vi "Demo.vi"() -> ()   [LabVIEW 2019]
uses:
  IO_VI/IOCtrl/Ctrl/IO Card_Type.ctl
panel:
  in  "IOType":enum16{"InputAndOutput", "Input", "OutPut"}(ring)
  in  "stop":bool
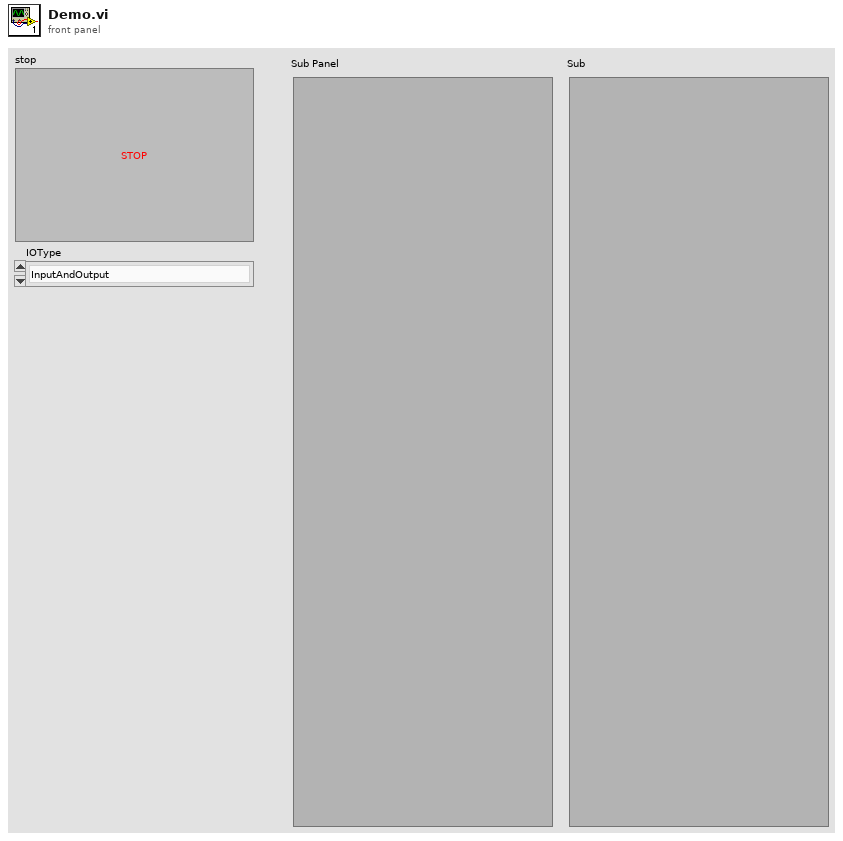
[diagram p1: front panel]
types:
  T1 = typedef "IO Card_Type.ctl" = enum16{"None", "Unidaq32", "6480", "2410C-64", "Zan", "DMC1000B"}
  T2 = typedef "LVPointTypeDef.ctl" = cluster{"Horizontal":i16, "Vertical":i16}
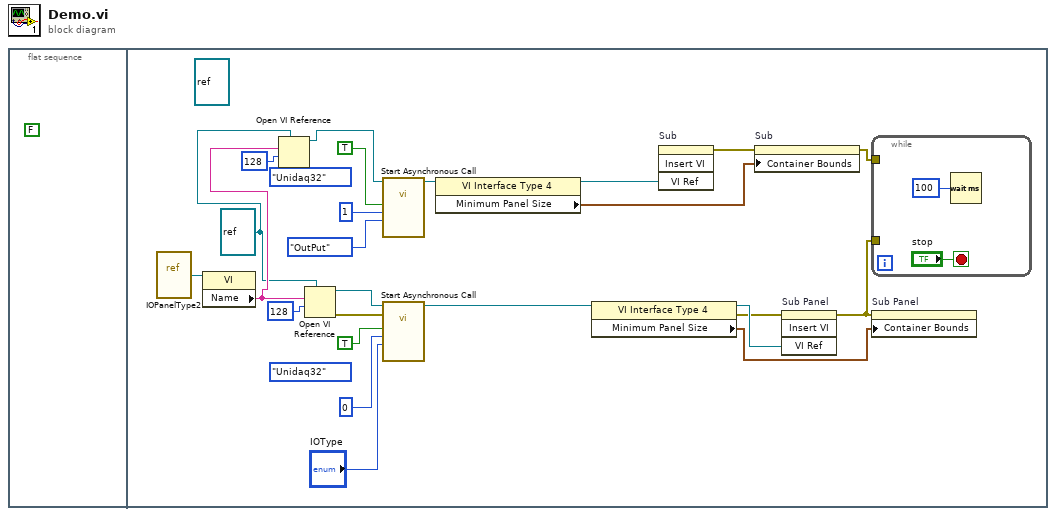
[diagram p0: block diagram]
diagram:
  n1 = flat-sequence {
    frame #0 {
      (unwired) FALSE ("Stopflg")
    }
    frame #1 {
      (unwired) refnum<vi> refnum ("reference out")
      (unwired) IO_Card_Type."Unidaq32" ("Card_Type")
      (unwired) IO_Card_Type."Unidaq32" ("Card_Type")
      w1 = refnum<vi> refnum ("reference out")
      n2 = vi-ref "IOPanelType2.vi"() -> (w23:refnum<vi>)
      n3 = property class="VI"(reference=w23) -> ("Name"=w3:string)  [unwired: 1 in, 2 out]
      n4 = Open VI Reference(type specifier VI Refnum (for type only)=w1, vi path=w3, options=128) -> (vi reference=w2:refnum<vi>)  [unwired: 3 in, 1 out]
      n5 = Open VI Reference(type specifier VI Refnum (for type only)=w1, vi path=w3, options=128) -> (vi reference=w5:refnum<vi>, error out=w19:errorcluster)  [unwired: 3 in]
      n6 = call-by-ref "Start Asynchronous Call"(reference=w2, "IOType"=enum16{"InputAndOutput", "Input", "OutPut"}."OutPut", "IOCardIndex"=u32 1, "insert"=TRUE) -> (reference out=w10:refnum<vi>)  [unwired: 10 in, 1 out]
      n7 = call-by-ref "Start Asynchronous Call"(reference=w5, error in=w19, "IOType"="IOType", "IOCardIndex"=u32 0, "insert"=TRUE) -> (reference out=w18:refnum<vi>)  [unwired: 9 in, 1 out]
      n8 = property class="VI Interface Type 4"(reference=w10) -> (reference out=w9:refnum<vi>, "Minimum Panel Size"=w8:T2)  [unwired: 1 in, 1 out]
      n9 = property class="VI Interface Type 4"(reference=w18) -> (reference out=w17:refnum<vi>, error out=w14:errorcluster, "Minimum Panel Size"=w16:T2)  [unwired: 1 in]
      n10 = invoke on="Sub" class="SubPnl" method="Insert VI"("VI Ref"=w9) -> (error out=w7:errorcluster)  [unwired: 3 in, 3 out]
      n11 = property on="Sub" class="SubPnl"(error in=w7, "Container Bounds"=w8) -> (error out=w6:errorcluster)  [unwired: 1 in, 1 out]
      n12 = invoke on="Sub Panel" class="SubPnl" method="Insert VI"(error in=w14, "VI Ref"=w17) -> (error out=w15:errorcluster)  [unwired: 2 in, 3 out]
      n13 = while {
        tunnel: w15 -> [_]
        tunnel: w6 -> [_]
        stop <- "stop" stop-if-true
        n14 = Wait (ms)(milliseconds to wait=u32 100 ("millisecond timer value")) -> ()  [unwired: 1 out]
      }
      n15 = property on="Sub Panel" class="SubPnl"(error in=w15, "Container Bounds"=w16) -> ()  [unwired: 1 in, 2 out]
    }
  }
